vi "Run.vi"(8 "error in (no error)":errorcluster, 9 "s on last turn":dbl, 10 "Maze (0: Empty, -1: Enemy. >0: Teammate":i32[][](array[numeric]), 11 "Scout In":refnum<class "Coward.lvclass">) -> (0 "error out":errorcluster, 1 "Direction":T1, 2 "Action":T2, 3 "Scout Out":refnum<class "Coward.lvclass">, 4 "Replicated":refnum<class "Runner.lvclass">)   [LabVIEW 2014, in "Coward.lvclass"]
uses:
  Coward.lvclass
  Action Enum.ctl
  Direction Enum.ctl
  Runner.lvclass
  Mother/Attack Options.ctl
  Coward.lvclass/Coward.ctl
  Mother/Mother.lvclass
  SquareBattle.lvclass
panel:
  in  "Status":string
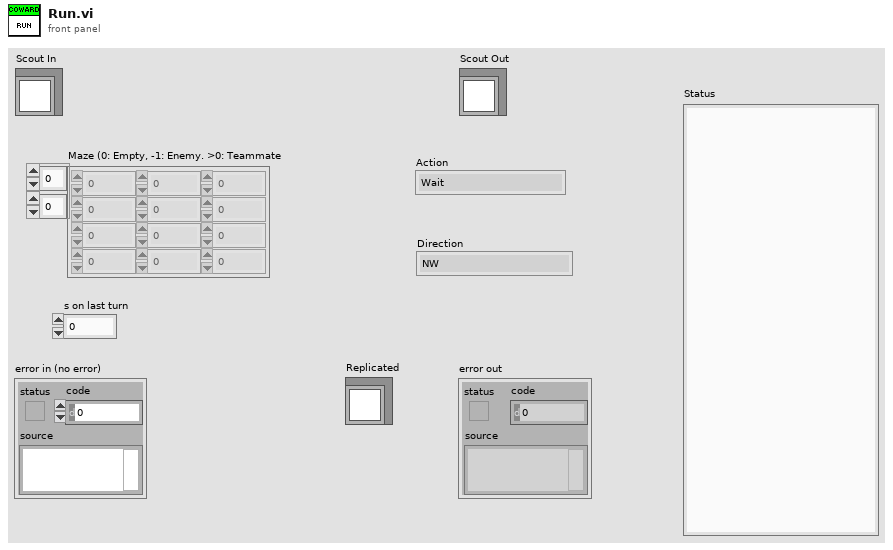
[diagram p1: front panel]
types:
  T1 = typedef "SquareBattle.lvclass/Direction Enum.ctl" = enum16{"NW", "N", "NE", "E", "SE", "S", "SW", "W"}
  T2 = typedef "SquareBattle.lvclass/Action Enum.ctl" = enum16{"Wait", "Move", "Attack", "Replicate"}
  T3 = typedef "Mother.lvclass/Attack Options.ctl" = enum16{"Attack", "Run", "Distract"}
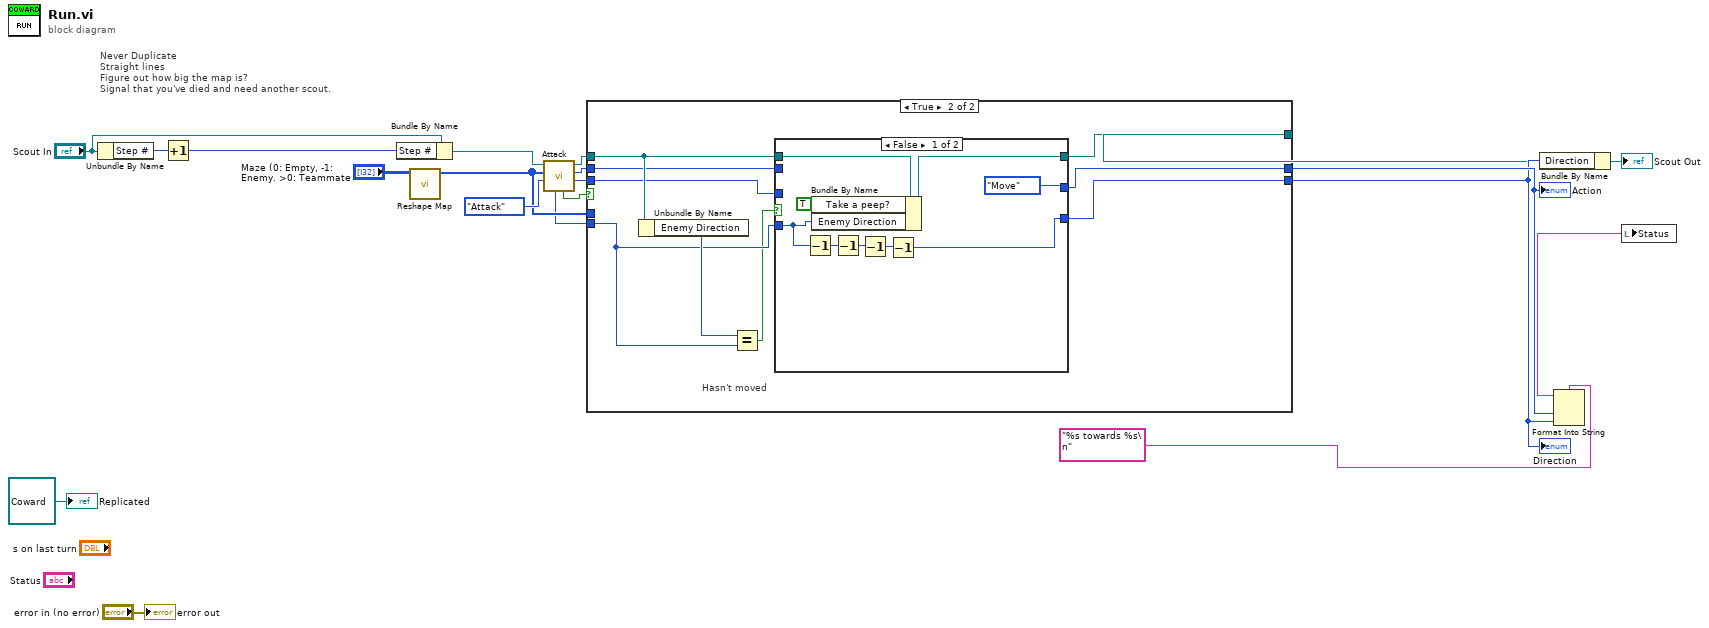
[diagram p0: block diagram]
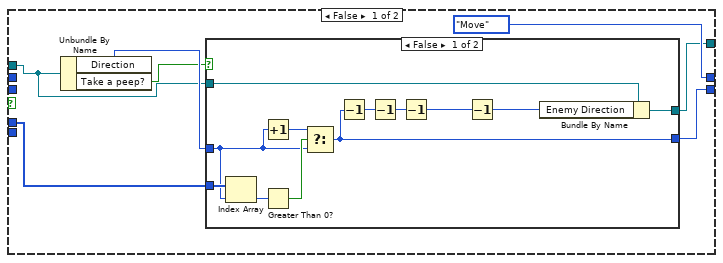
[diagram p2: hidden frame]
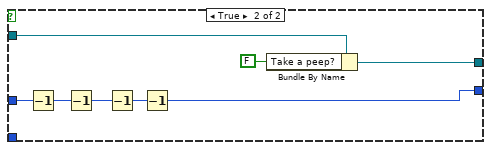
[diagram p3: hidden frame]
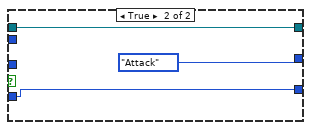
[diagram p4: hidden frame]
diagram:
  # "Never Duplicate\nStraight lines\nFigure out how big the map is?\nSignal that you've died and need another scout."
  n1 = Unbundle By Name("Scout In") -> ("Step #"=w5:i32)
  n2 = Increment(x=w5) -> (x+1=w17:i32)
  n3 = Bundle By Name(cluster="Scout In", "Step #"=w17) -> (w15:refnum<class "Coward.lvclass">)
  n4 = call "Reshape Map.vi"("Maze (0: Empty, -1: Enemy. >0: Teammate"="Maze (0: Empty, -1: Enemy. >0: Teammate") -> ("Map"=w4:i32[])  [unwired: 9 in, 1 out]
  n5 = call "Attack.vi"("Attack?"=Attack_Options."Attack", "Maze (0: Empty, -1: Enemy. >0: Teammate"=w4, "Mother in"=w15) -> ("Direction"=w9:T1, "Action"=w11:T2, "Mother out"=w3:refnum<class "Coward.lvclass">, "Enemy Found?"=w12:bool, "Enemy Direction"=w1:T1)  [unwired: 3 in, 1 out]
  n6 = case shown="True" w12 {
    tunnel: w11 -> [_ w53]
    tunnel: [Action_Enum."Move" ("Action") w52] -> w10
    tunnel: w9 -> [_ w54]
    tunnel: [w26 w51] -> w8
    tunnel: w4 -> [w25 _]
    tunnel: w3 -> [w22 w55]
    tunnel: [w21 w56] -> w2
    tunnel: w1 -> [_ w49]
    frame False {
      n7 = Unbundle By Name(w22) -> ("Direction"=w24:T1, "Take a peep?"=w23:bool)
      n8 = case shown="False" w23 {
        tunnel: [w32 w43] -> w26
        tunnel: w25 -> [w39 _]
        tunnel: w24 -> [w35 w47]
        tunnel: w22 -> [w34 w42]
        tunnel: [w33 w41] -> w21
        frame False {
          n9 = Index Array(array=w39, index=w35) -> (element=w38:i32)
          n10 = Increment(x=w35) -> (x+1=w36:T1)
          n11 = Greater Than 0?(x=w38) -> (x > 0?=w37:bool)
          n12 = Select(t=w36, s=w37, f=w35) -> (s? t:f=w32:T1)
          n13 = Decrement(x=w32) -> (x-1=w31:T1)
          n14 = Decrement(x=w31) -> (x-1=w30:T1)
          n15 = Decrement(x=w30) -> (x-1=w29:T1)
          n16 = Decrement(x=w29) -> (x-1=w28:T1)
          n17 = Bundle By Name(cluster=w34, "Enemy Direction"=w28) -> (w33:refnum<class "Coward.lvclass">)
        }
        frame True {
          n18 = Decrement(x=w47) -> (x-1=w46:T1)
          n19 = Decrement(x=w46) -> (x-1=w45:T1)
          n20 = Decrement(x=w45) -> (x-1=w44:T1)
          n21 = Decrement(x=w44) -> (x-1=w43:T1)
          n22 = Bundle By Name(cluster=w42, "Take a peep?"=FALSE) -> (w41:refnum<class "Coward.lvclass">)
        }
      }
    }
    frame True {
      # "Hasn't moved"
      n23 = Unbundle By Name(w55) -> ("Enemy Direction"=w50:T1)
      n24 = Equal?(x=w50, y=w49) -> (x = y?=w48:bool)
      n25 = case shown="False" w48 {
        tunnel: [w65 w68] -> w56
        tunnel: w55 -> [w63 w68]
        tunnel: w54 -> [_ _]
        tunnel: w53 -> [_ _]
        tunnel: [Action_Enum."Move" ("Action") Action_Enum."Attack" ("Action")] -> w52
        tunnel: [w58 w66] -> w51
        tunnel: w49 -> [w59 w66]
        frame False {
          n26 = Decrement(x=w59) -> (x-1=w62:T1)
          n27 = Bundle By Name(cluster=w63, "Take a peep?"=TRUE, "Enemy Direction"=w59) -> (w65:refnum<class "Coward.lvclass">)
          n28 = Decrement(x=w62) -> (x-1=w60:T1)
          n29 = Decrement(x=w60) -> (x-1=w61:T1)
          n30 = Decrement(x=w61) -> (x-1=w58:T1)
        }
        frame True {
        }
      }
    }
  }
  "Action" <- w10
  "Direction" <- w8
  n31 = Bundle By Name(cluster=w2, "Direction"=w8) -> (→"Scout Out":refnum<class "Coward.lvclass">)
  n32 = Format Into String(format string="%s towards %s\n", w10, w8) -> (resulting string=w6:string)  [unwired: 2 in, 1 out]
  n33 = local write "Status"(w6) -> ()
  "error out" <- "error in (no error)"
  "Replicated" <- refnum<class "Coward.lvclass"> refnum ("Replicated")
